vi "GetFolderSizeInBytes.vi"(8 "error in (no error)":errorcluster, 11 "Folder":path) -> (0 "error out":errorcluster, 3 "FolderSize (bytes)":i64)   [LabVIEW 2015, in "TronviewGame.lvlib" / "Game.lvclass"]
uses:
  Game.lvclass
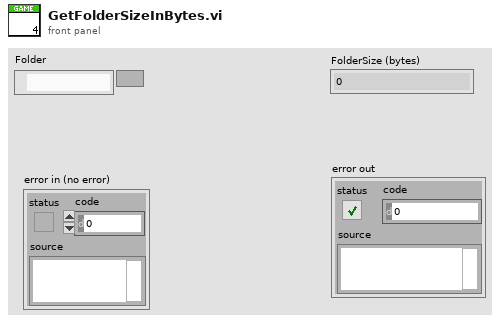
[diagram p1: front panel]
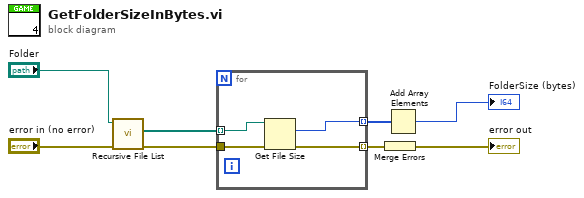
[diagram p0: block diagram]
diagram:
  n1 = call <vilib>:"Recursive File List.vi"("error in (no error)"="error in (no error)", "Folder Path"="Folder") -> ("error out"=w3:errorcluster, "All Files in Dir"=w7:path[])  [unwired: 5 in, 3 out]
  n2 = for {
    tunnel: w7 -> [w12] mode=indexing
    tunnel: [w11] -> w6 mode=indexing
    tunnel: w3 -> [w10]
    tunnel: [w9] -> w2 mode=indexing
    n3 = Get File Size(file=w12, error in=w10) -> (size (in bytes)=w11:i64, 0:w9:errorcluster)  [unwired: 1 out]
  }
  n4 = Merge Errors(w2) -> (→"error out":errorcluster)
  n5 = Add Array Elements(numeric array=w6) -> (sum=→"FolderSize (bytes)":i64)
